vi "Tag Engine Test 2.vi"() -> ()   [LabVIEW 2020]
doc: "_Test_"
uses:
  Tag/Tag.lvclass
  Tag/Tag.lvclass/Tag.ctl
  Core/Tag Core.lvclass/Tag Core.ctl
  3d4b882a-e436-4f37-aed9-35a305ddb346.vi
  eb00c9cd-5161-4d26-ae32-490fe508d5fe.vi
  73cf2a16-35a3-43c1-b628-a6dee5632637.vi
  77c790be-6133-48fa-abcc-627f330f8da1.vi
  0c08567f-0fa1-42bb-8d57-fa012ad98f57.vi
  8b0f5b2c-ae71-4c49-821c-81fbe44761c9.vi
  42aa8062-1980-4d59-a8f6-0165d054f103.vi
  437add60-3501-4199-a226-20a01a6dbd58.vi
  fbc51c97-2a17-48fa-b791-483b54fb73e8.vi
  2fe9b505-b9e1-4519-be3b-b52b5f1ea9e9.vi
  17b4772d-3788-4d19-9513-47d70780018f.vi
  Tag/Construct.vi
  Core/Write Tag Value_ByRef.vi
  Core/Get Tag.vi
  Core/Get Tag Value_ByRef.vi
  Tools/SubVIs/Array of VData to VCluster_openG.vi
  Tag/Write Value with Timestamp.vi
  Tag/Read Value.vi
  Tag/Read Timestamp.vi
  Tag/Set Properties from Initial.vi
  Core/Add Tag.vi
  Core/Get Tag LUT.vi
  <vilib>/Utility/error.llb/Error Cluster From Error Code.vi
  <vilib>/Utility/Data Type/Get Type Information.vi
  <vilib>/JDP Science/JSONtext/Variant to JSON Text.vi
  <vilib>/Utility/Data Type/Get Cluster Information.vi
  Tag Engine.lvlib
panel:
  out "error out":errorcluster
  out "Value 3":dbl
  out "Timestamp":timestamp[](array[timestamp])
  out "Value 2":variant[](array[variant])
  out "Value":string[](array[string])
  out "error out 3":errorcluster
  out "Write":dbl=42.0
  out "Pass 3":bool caption="Write Multiple Same Value"
  out "error out 1":errorcluster
  out "Pass 2":bool caption="Write Multiple by Ref Pass"
  out "Pass 1":bool caption="Write Multiple by Name Pass"
  out "Read":dbl[](array[numeric])
  out "Array 2":string[](array[string])=["GROUP1:TAG1", "GROUP1:TAG2", "GROUP1:TAG3", "GROUP1:TAG4"]
  out "error out 2":errorcluster
  out "Read by Ref":dbl[](array[numeric])
  out "Write by Ref":dbl[](array[numeric])
  out "Write by Name":dbl[](array[numeric])
  out "Read by Name":dbl[](array[numeric])
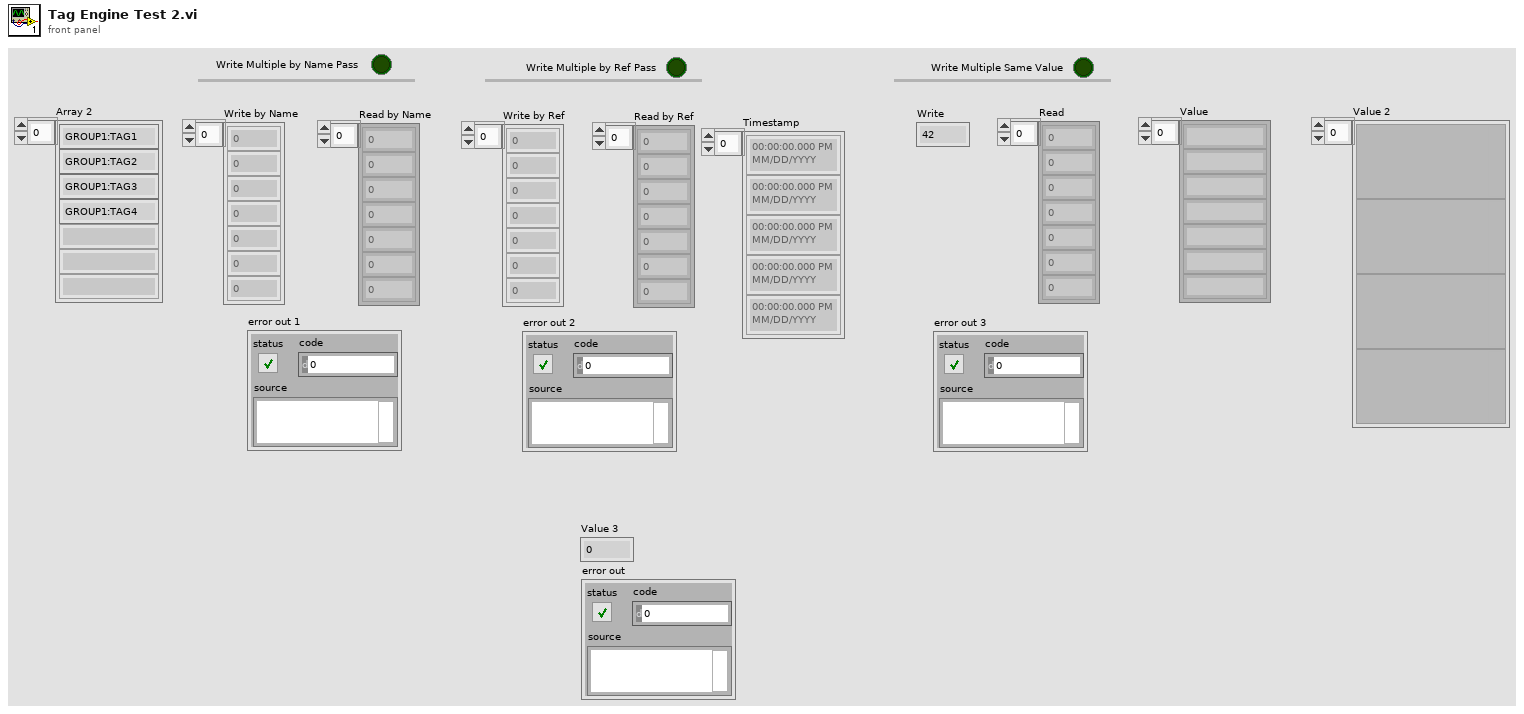
[diagram p1: front panel]
types:
  T1 = cluster{"TAG1":refnum<data-value>, "TAG2":refnum<data-value>, "TAG3":refnum<data-value>}
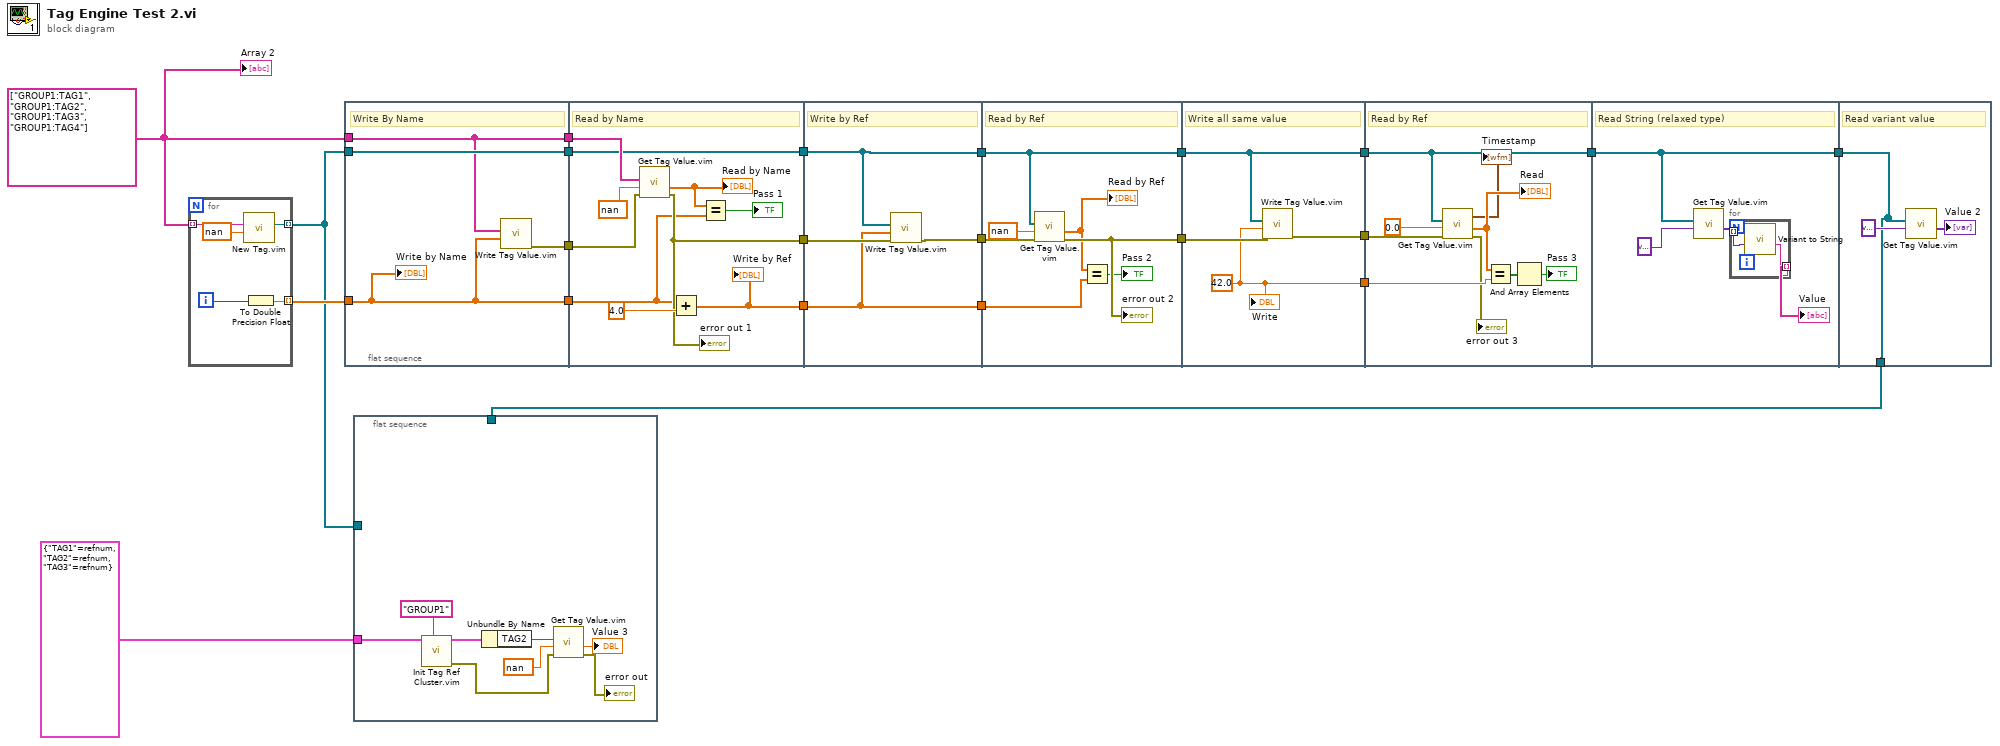
[diagram p0: block diagram]
diagram:
  w22 = string[] ["GROUP1:TAG1", "GROUP1:TAG2", "GROUP1:TAG3", "GROUP1:TAG4"]
  n1 = for {
    tunnel: w22 -> [w27] mode=indexing
    tunnel: [w25] -> w3 mode=indexing
    tunnel: [w23] -> w21 mode=indexing
    i -> [w24]
    n2 = call "New Tag.vim"("Initial Value"=nan, "Tag Name"=w27) -> ("Tag Ref out"=w25:refnum<data-value>)  [unwired: 8 in, 1 out]
    n3 = To Double Precision Float(number=w24) -> (double precision float=w23:dbl)
  }
  n4 = flat-sequence {
    tunnel: w22 -> [w30]
    tunnel: w3 -> [w31]
    tunnel: w21 -> [w29]
    tunnel: [w30] -> w20
    tunnel: [w29] -> w19
    tunnel: [w31] -> w16
    tunnel: [w28] -> w12
    tunnel: w20 -> [w41]
    tunnel: w19 -> [w33]
    tunnel: [w38] -> w18
    tunnel: [w37] -> w17
    tunnel: w16 -> [w37]
    tunnel: [w36] -> w13
    tunnel: w12 -> [w35]
    tunnel: w18 -> [w42]
    tunnel: w17 -> [w45]
    tunnel: [w45] -> w15
    tunnel: [w44] -> w14
    tunnel: w13 -> [w43]
    tunnel: [w42] -> w7
    tunnel: w15 -> [w50]
    tunnel: w14 -> [w51]
    tunnel: [w50] -> w11
    tunnel: [w49] -> w10
    tunnel: w7 -> [w46]
    tunnel: w11 -> [w54]
    tunnel: w10 -> [w56]
    tunnel: [w55] -> w9
    tunnel: [w54] -> w8
    tunnel: [w53] -> w6
    tunnel: w9 -> [w65]
    tunnel: w8 -> [w58]
    tunnel: w6 -> [w63]
    tunnel: [w58] -> w5
    tunnel: w5 -> [w69]
    tunnel: [w69] -> w4
    tunnel: w4 -> [w72]
    tunnel: [w72] -> w1
    frame #0 {
      # "Write By Name"
      n5 = call "Write Tag Value.vim"("Value"=w29, "Tag Name(s)/Ref(s)"=w30) -> ("error out"=w28:errorcluster)  [unwired: 8 in, 1 out]
      "Write by Name" <- w29
    }
    frame #1 {
      # "Read by Name"
      n6 = call "Get Tag Value.vim"("error in (no error)"=w35, "Default (Void)"=nan, "Tag Name(s)/Ref(s)"=w41) -> ("error out"=w36:errorcluster, "Value(s)"=w34:dbl[])  [unwired: 5 in, 2 out]
      "Read by Name" <- w34
      "error out 1" <- w36
      n7 = Add(x=w33, y=4.0) -> (x+y=w38:dbl[])
      "Write by Ref" <- w38
      n8 = Equal?(x=w34, y=w33) -> (x = y?=→"Pass 1":bool)
    }
    frame #2 {
      # "Write by Ref"
      n9 = call "Write Tag Value.vim"("error in (no error)"=w43, "Value"=w42, "Tag Name(s)/Ref(s)"=w45) -> ("error out"=w44:errorcluster)  [unwired: 7 in, 1 out]
    }
    frame #3 {
      # "Read by Ref"
      n10 = call "Get Tag Value.vim"("error in (no error)"=w51, "Default (Void)"=nan, "Tag Name(s)/Ref(s)"=w50) -> ("error out"=w49:errorcluster, "Value(s)"=w47:dbl[])  [unwired: 5 in, 2 out]
      "Read by Ref" <- w47
      "error out 2" <- w49
      n11 = Equal?(x=w47, y=w46) -> (x = y?=→"Pass 2":bool)
    }
    frame #4 {
      w53 = 42.0
      # "Write all same value"
      n12 = call "Write Tag Value.vim"("error in (no error)"=w56, "Value"=w53, "Tag Name(s)/Ref(s)"=w54) -> ("error out"=w55:errorcluster)  [unwired: 7 in, 1 out]
      "Write" <- w53
    }
    frame #5 {
      # "Read by Ref"
      n13 = call "Get Tag Value.vim"("error in (no error)"=w65, "Default (Void)"=0.0, "Tag Name(s)/Ref(s)"=w58) -> ("error out"=→"error out 3":errorcluster, "Value(s)"=w62:dbl[], "Timestamp(s)"=→"Timestamp":timestamp[])  [unwired: 5 in, 1 out]
      "Read" <- w62
      n14 = Equal?(x=w62, y=w63) -> (x = y?=w61:bool[])
      n15 = And Array Elements(Boolean array=w61) -> (logical AND=→"Pass 3":bool)
    }
    frame #6 {
      # "Read String (relaxed type)"
      n16 = call "Get Tag Value.vim"("Default (Void)"=variant, "Tag Name(s)/Ref(s)"=w69) -> ("Value(s)"=w67:variant[])  [unwired: 6 in, 3 out]
      n17 = for {
        tunnel: w67 -> [w71] mode=indexing
        tunnel: [w70] -> w66 mode=indexing
        n18 = call "Variant to String.vi"("Variant Value"=w71) -> ("String Value"=w70:string)  [unwired: 9 in, 1 out]
      }
      "Value" <- w66
    }
    frame #7 {
      # "Read variant value"
      n19 = call "Get Tag Value.vim"("Default (Void)"=variant, "Tag Name(s)/Ref(s)"=w72) -> ("Value(s)"=→"Value 2":variant[])  [unwired: 6 in, 3 out]
    }
  }
  n20 = flat-sequence {
    tunnel: w3 -> [_]
    tunnel: T1 {"TAG1"=refnum, "TAG2"=refnum, "TAG3"=refnum} -> [w82]
    tunnel: w1 -> [_]
    frame #0 {
      n21 = call "Init Tag Ref Cluster.vim"("Namespace"="GROUP1", "Tag Refs in"=w82) -> ("error out"=w76:errorcluster, "Tag Refs out"=w80:T1)  [unwired: 7 in, 1 out]
      n22 = Unbundle By Name(w80) -> ("TAG2"=w79:refnum<data-value>)
      n23 = call "Get Tag Value.vim"("error in (no error)"=w76, "Default (Void)"=nan, "Tag Name(s)/Ref(s)"=w79) -> ("error out"=→"error out":errorcluster, "Value(s)"=→"Value 3":dbl)  [unwired: 5 in, 2 out]
    }
  }
  "Array 2" <- w22
